vi "VI Tree.vi"   [LabVIEW 2020, in "Agilent 90000 Series.lvlib"]
doc: "This is the instrument driver for the Agilent 90000 and 9000 Series Oscilloscopes. The VI Tree displays all the user-callable VIs of the instrument driver in an organized table."
uses:
  Agilent 90000 Series.lvlib
  Configure/IScan/Configure IScan Trigger (Measurement Limit).vi
  Configure/Measurement/Configure Measurement (Burst Width).vi
  Configure/Trigger/Configure Trigger (Communication).vi
  Data/Read and Save as TDMS (Single Channel).vi
  Data/Read Waveform from TDMS (Unscaled Int8).vi
  Data/Read (Multiple Digital Waveforms).vi
  Data/Low Level/Fetch Measurement (Burst Interval).vi
  Data/Low Level/Fetch (Digital Waveform).vi
  Configure/Measurement/Configure Measurement Characteristics (Eye Pattern).vi
  Data/Read Measurement (Burst Interval).vi
  Configure/Configure Math (Binary Operation).vi
panel:
  # "(c) 2011-2014 National Instruments.  ALL RIGHTS RESERVED."
  # "SEE DIAGRAM\nFOR VI TREE."
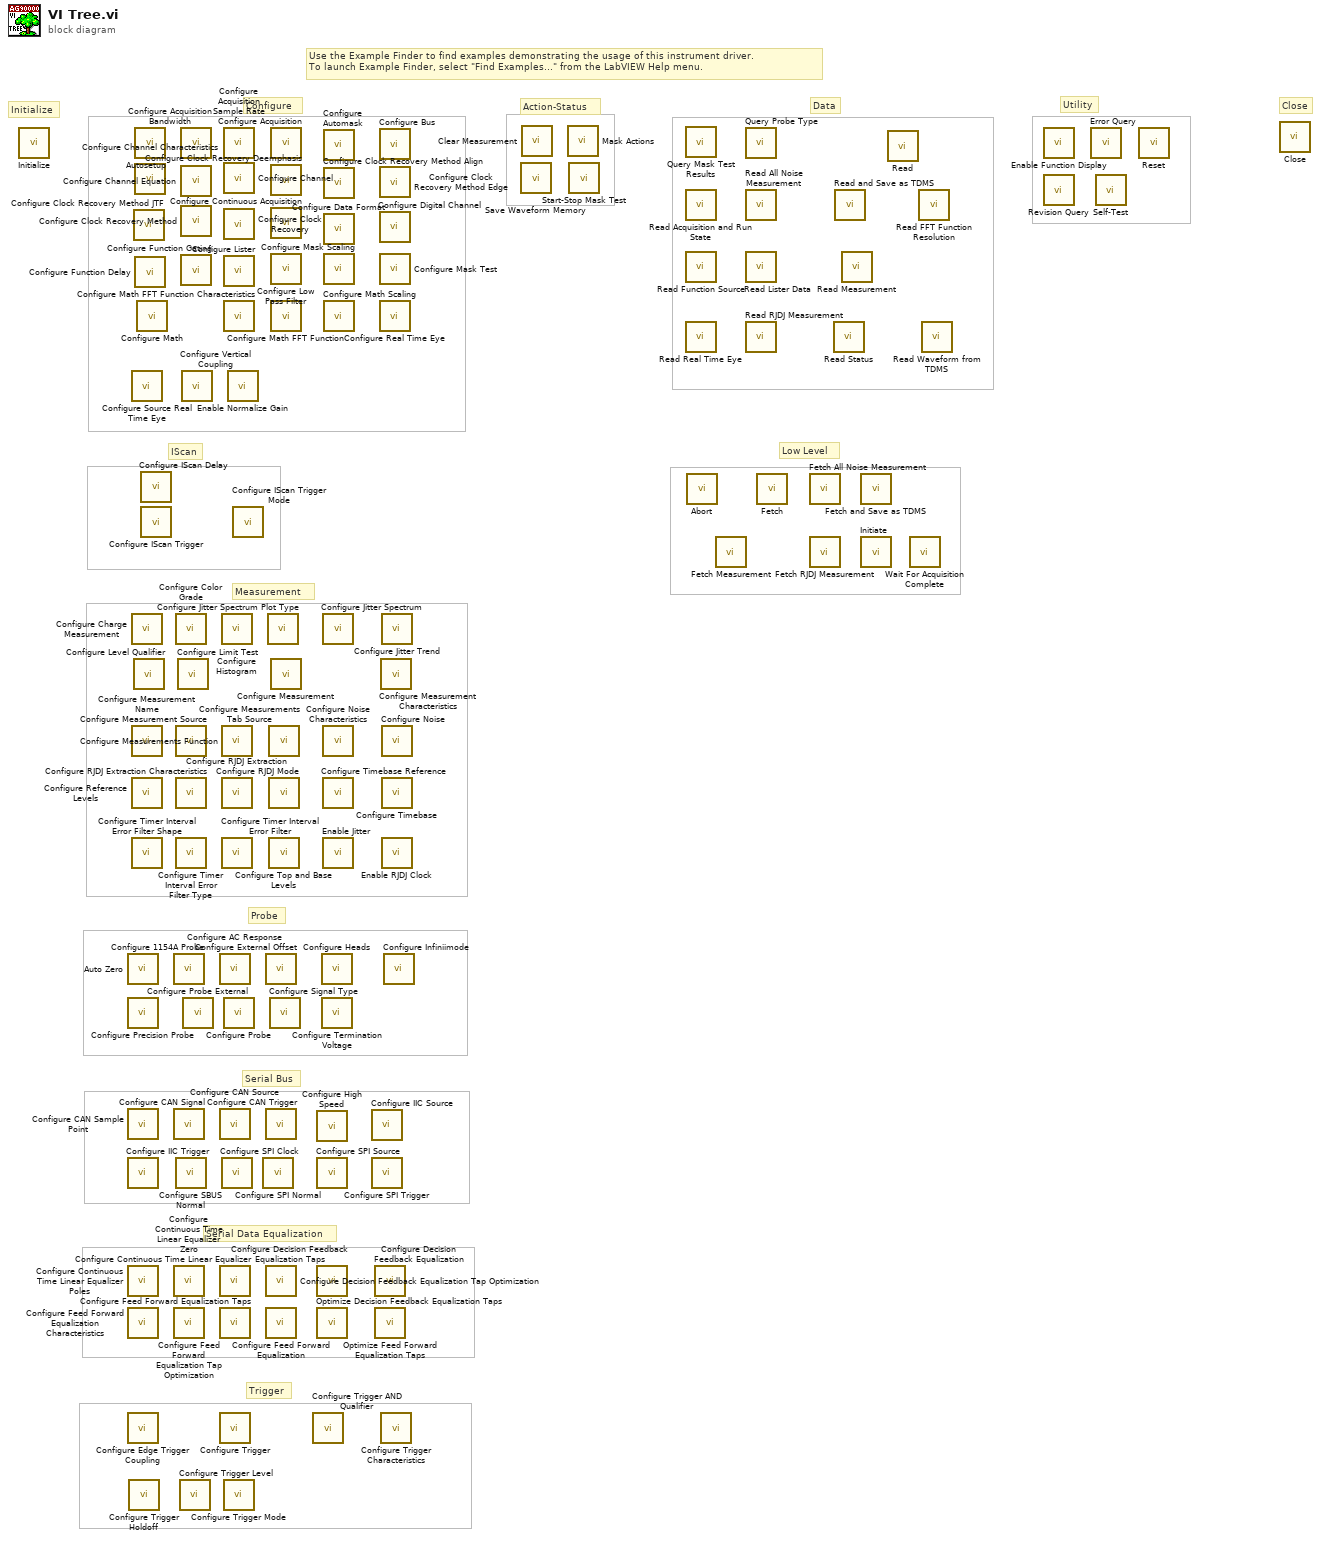
[diagram p0: block diagram]
diagram:
  # "Close"
  # "Utility"
  # "Low Level"
  # "Data"
  # "Trigger"
  # "Serial Data Equalization"
  # "Serial Bus"
  # "Probe"
  # "Measurement"
  # "IScan"
  # "Configure"
  # "Action-Status"
  # "Initialize"
  # "Use the Example Finder to find examples demonstrating the usage of this instrument driver.\nTo launch Example Finder, select \"Find Examples...\" from the LabVIEW Help menu."
  n1 = call "Initialize.vi"() -> ()  [unwired: 9 in, 3 out]
  n2 = call "Auto Zero.vi"() -> ()  [unwired: 10 in, 2 out]
  n3 = call "Configure Precision Probe.vi"() -> ()  [unwired: 14 in, 2 out]
  n4 = call "Configure CAN Sample Point.vi"() -> ()  [unwired: 10 in, 2 out]
  n5 = call "Configure IIC Trigger.vi"() -> ()  [unwired: 10 in, 2 out]
  n6 = call "Configure Continuous Time Linear Equalizer Poles.vi"() -> ()  [unwired: 10 in, 2 out]
  n7 = call "Configure Feed Forward Equalization Characteristics.vi"() -> ()  [unwired: 10 in, 2 out]
  n8 = call "Configure Edge Trigger Coupling.vi"() -> ()  [unwired: 14 in, 2 out]
  n9 = call "Configure Trigger Holdoff.vi"() -> ()  [unwired: 10 in, 2 out]
  n10 = call "Configure Source Real Time Eye.vi"() -> ()  [unwired: 10 in, 2 out]
  n11 = call "Configure Charge Measurement.vi"() -> ()  [unwired: 10 in, 2 out]
  n12 = call "Configure Measurement Name.vi"() -> ()  [unwired: 10 in, 2 out]
  n13 = call "Configure Reference Levels.vi"() -> ()  [unwired: 10 in, 2 out]
  n14 = call "Configure Timer Interval Error Filter Shape.vi"() -> ()  [unwired: 10 in, 2 out]
  n15 = call "Configure Clock Recovery Method JTF.vi"() -> ()  [unwired: 14 in, 2 out]
  n16 = call "Configure Level Qualifier.vi"() -> ()  [unwired: 10 in, 2 out]
  n17 = call "Autosetup.vi"() -> ()  [unwired: 10 in, 2 out]
  n18 = call "Configure Channel Characteristics.vi"() -> ()  [unwired: 10 in, 2 out]
  n19 = call "Configure Function Delay.vi"() -> ()  [unwired: 10 in, 2 out]
  n20 = call-poly "Configure Math.vi"() -> ()  [unwired: 14 in, 2 out]
  n21 = call "Configure IScan Delay.vi"() -> ()  [unwired: 10 in, 2 out]
  n22 = call-poly "Configure IScan Trigger.vi"() -> ()  [unwired: 14 in, 2 out]
  n23 = call "Configure 1154A Probe.vi"() -> ()  [unwired: 10 in, 2 out]
  n24 = call "Configure CAN Signal.vi"() -> ()  [unwired: 10 in, 2 out]
  n25 = call "Configure Continuous Time Linear Equalizer Zero.vi"() -> ()  [unwired: 10 in, 2 out]
  n26 = call "Configure Feed Forward Equalization Tap Optimization.vi"() -> ()  [unwired: 10 in, 2 out]
  n27 = call "Configure Color Grade.vi"() -> ()  [unwired: 14 in, 2 out]
  n28 = call "Configure Measurement Source.vi"() -> ()  [unwired: 10 in, 2 out]
  n29 = call "Configure RJDJ Extraction Characteristics.vi"() -> ()  [unwired: 14 in, 2 out]
  n30 = call "Configure Timer Interval Error Filter Type.vi"() -> ()  [unwired: 14 in, 2 out]
  n31 = call "Configure SBUS Normal.vi"() -> ()  [unwired: 10 in, 2 out]
  n32 = call "Configure Limit Test.vi"() -> ()  [unwired: 10 in, 2 out]
  n33 = call "Configure Trigger Level.vi"() -> ()  [unwired: 10 in, 2 out]
  n34 = call "Configure Acquisition Bandwidth.vi"() -> ()  [unwired: 10 in, 2 out]
  n35 = call "Configure Channel Equation.vi"() -> ()  [unwired: 10 in, 2 out]
  n36 = call "Configure Clock Recovery Method.vi"() -> ()  [unwired: 14 in, 2 out]
  n37 = call "Configure Function Gating.vi"() -> ()  [unwired: 10 in, 2 out]
  n38 = call "Configure Vertical Coupling.vi"() -> ()  [unwired: 10 in, 2 out]
  n39 = call "Configure Probe External.vi"() -> ()  [unwired: 10 in, 2 out]
  n40 = call "Configure AC Response.vi"() -> ()  [unwired: 10 in, 2 out]
  n41 = call "Configure CAN Source.vi"() -> ()  [unwired: 10 in, 2 out]
  n42 = call "Configure Continuous Time Linear Equalizer.vi"() -> ()  [unwired: 14 in, 2 out]
  n43 = call "Configure Feed Forward Equalization Taps.vi"() -> ()  [unwired: 10 in, 2 out]
  n44 = call-poly "Configure Trigger.vi"() -> ()  [unwired: 14 in, 2 out]
  n45 = call "Configure Histogram.vi"() -> ()  [unwired: 14 in, 2 out]
  n46 = call "Configure Measurements Function.vi"() -> ()  [unwired: 10 in, 2 out]
  n47 = call "Configure RJDJ Extraction.vi"() -> ()  [unwired: 14 in, 2 out]
  n48 = call "Configure Timer Interval Error Filter.vi"() -> ()  [unwired: 14 in, 2 out]
  n49 = call "Configure SPI Clock.vi"() -> ()  [unwired: 10 in, 2 out]
  n50 = call "Configure Acquisition Sample Rate.vi"() -> ()  [unwired: 10 in, 2 out]
  n51 = call "Configure Channel.vi"() -> ()  [unwired: 10 in, 2 out]
  n52 = call "Configure Clock Recovery.vi"() -> ()  [unwired: 10 in, 2 out]
  n53 = call "Configure Lister.vi"() -> ()  [unwired: 10 in, 2 out]
  n54 = call "Configure Math FFT Function Characteristics.vi"() -> ()  [unwired: 10 in, 2 out]
  n55 = call "Configure Probe.vi"() -> ()  [unwired: 10 in, 2 out]
  n56 = call "Configure Trigger Mode.vi"() -> ()  [unwired: 14 in, 2 out]
  n57 = call "Enable Normalize Gain.vi"() -> ()  [unwired: 10 in, 2 out]
  n58 = call "Configure IScan Trigger Mode.vi"() -> ()  [unwired: 10 in, 2 out]
  n59 = call "Configure SPI Normal.vi"() -> ()  [unwired: 10 in, 2 out]
  n60 = call "Configure External Offset.vi"() -> ()  [unwired: 10 in, 2 out]
  n61 = call "Configure CAN Trigger.vi"() -> ()  [unwired: 14 in, 2 out]
  n62 = call "Configure Decision Feedback Equalization Tap Optimization.vi"() -> ()  [unwired: 10 in, 2 out]
  n63 = call "Configure Feed Forward Equalization.vi"() -> ()  [unwired: 14 in, 2 out]
  n64 = call "Configure Jitter Spectrum Plot Type.vi"() -> ()  [unwired: 10 in, 2 out]
  n65 = call "Configure Measurements Tab Source.vi"() -> ()  [unwired: 10 in, 2 out]
  n66 = call "Configure RJDJ Mode.vi"() -> ()  [unwired: 10 in, 2 out]
  n67 = call "Configure Top and Base Levels.vi"() -> ()  [unwired: 14 in, 2 out]
  n68 = call "Configure Signal Type.vi"() -> ()  [unwired: 10 in, 2 out]
  n69 = call "Configure Acquisition.vi"() -> ()  [unwired: 14 in, 2 out]
  n70 = call "Configure Clock Recovery Deemphasis.vi"() -> ()  [unwired: 10 in, 2 out]
  n71 = call "Configure Continuous Acquisition.vi"() -> ()  [unwired: 10 in, 2 out]
  n72 = call "Configure Low Pass Filter.vi"() -> ()  [unwired: 10 in, 2 out]
  n73 = call "Configure Math FFT Function.vi"() -> ()  [unwired: 10 in, 2 out]
  n74 = call-poly "Configure Measurement.vi"() -> ()  [unwired: 14 in, 2 out]
  n75 = call "Configure Trigger AND Qualifier.vi"() -> ()  [unwired: 14 in, 2 out]
  n76 = call "Configure High Speed.vi"() -> ()  [unwired: 14 in, 2 out]
  n77 = call "Configure SPI Source.vi"() -> ()  [unwired: 10 in, 2 out]
  n78 = call "Configure Decision Feedback Equalization Taps.vi"() -> ()  [unwired: 10 in, 2 out]
  n79 = call "Optimize Decision Feedback Equalization Taps.vi"() -> ()  [unwired: 10 in, 2 out]
  n80 = call "Configure Heads.vi"() -> ()  [unwired: 10 in, 2 out]
  n81 = call "Configure Termination Voltage.vi"() -> ()  [unwired: 10 in, 2 out]
  n82 = call "Configure Jitter Spectrum.vi"() -> ()  [unwired: 14 in, 2 out]
  n83 = call "Configure Noise Characteristics.vi"() -> ()  [unwired: 10 in, 2 out]
  n84 = call "Configure Timebase Reference.vi"() -> ()  [unwired: 10 in, 2 out]
  n85 = call "Enable Jitter.vi"() -> ()  [unwired: 10 in, 2 out]
  n86 = call "Configure Automask.vi"() -> ()  [unwired: 10 in, 2 out]
  n87 = call "Configure Clock Recovery Method Align.vi"() -> ()  [unwired: 10 in, 2 out]
  n88 = call "Configure Data Format.vi"() -> ()  [unwired: 10 in, 2 out]
  n89 = call "Configure Mask Scaling.vi"() -> ()  [unwired: 10 in, 2 out]
  n90 = call "Configure Math Scaling.vi"() -> ()  [unwired: 10 in, 2 out]
  n91 = call "Configure IIC Source.vi"() -> ()  [unwired: 10 in, 2 out]
  n92 = call "Configure SPI Trigger.vi"() -> ()  [unwired: 10 in, 2 out]
  n93 = call "Configure Decision Feedback Equalization.vi"() -> ()  [unwired: 14 in, 2 out]
  n94 = call "Optimize Feed Forward Equalization Taps.vi"() -> ()  [unwired: 10 in, 2 out]
  n95 = call "Configure Bus.vi"() -> ()  [unwired: 10 in, 2 out]
  n96 = call "Configure Clock Recovery Method Edge.vi"() -> ()  [unwired: 10 in, 2 out]
  n97 = call "Configure Digital Channel.vi"() -> ()  [unwired: 10 in, 2 out]
  n98 = call "Configure Mask Test.vi"() -> ()  [unwired: 14 in, 2 out]
  n99 = call "Configure Real Time Eye.vi"() -> ()  [unwired: 14 in, 2 out]
  n100 = call-poly "Configure Measurement Characteristics.vi"() -> ()  [unwired: 14 in, 2 out]
  n101 = call "Configure Trigger Characteristics.vi"() -> ()  [unwired: 14 in, 2 out]
  n102 = call "Configure Jitter Trend.vi"() -> ()  [unwired: 14 in, 2 out]
  n103 = call "Configure Noise.vi"() -> ()  [unwired: 10 in, 2 out]
  n104 = call "Configure Timebase.vi"() -> ()  [unwired: 10 in, 2 out]
  n105 = call "Enable RJDJ Clock.vi"() -> ()  [unwired: 10 in, 2 out]
  n106 = call "Configure Infiniimode.vi"() -> ()  [unwired: 10 in, 2 out]
  n107 = call "Save Waveform Memory.vi"() -> ()  [unwired: 10 in, 2 out]
  n108 = call "Clear Measurement.vi"() -> ()  [unwired: 10 in, 2 out]
  n109 = call "Mask Actions.vi"() -> ()  [unwired: 10 in, 2 out]
  n110 = call "Start-Stop Mask Test.vi"() -> ()  [unwired: 10 in, 2 out]
  n111 = call "Query Mask Test Results.vi"() -> ()  [unwired: 6 in, 6 out]
  n112 = call "Read Acquisition and Run State.vi"() -> ()  [unwired: 8 in, 4 out]
  n113 = call "Read Function Source.vi"() -> ()  [unwired: 8 in, 4 out]
  n114 = call "Read Real Time Eye.vi"() -> ()  [unwired: 8 in, 4 out]
  n115 = call "Abort.vi"() -> ()  [unwired: 10 in, 2 out]
  n116 = call-poly "Fetch Measurement.vi"() -> ()  [unwired: 13 in, 3 out]
  n117 = call "Query Probe Type.vi"() -> ()  [unwired: 9 in, 3 out]
  n118 = call "Read All Noise Measurement.vi"() -> ()  [unwired: 6 in, 10 out]
  n119 = call "Read Lister Data.vi"() -> ()  [unwired: 9 in, 3 out]
  n120 = call "Read RJDJ Measurement.vi"() -> ()  [unwired: 5 in, 11 out]
  n121 = call-poly "Fetch.vi"() -> ()  [unwired: 13 in, 3 out]
  n122 = call "Fetch All Noise Measurement.vi"() -> ()  [unwired: 6 in, 10 out]
  n123 = call "Fetch RJDJ Measurement.vi"() -> ()  [unwired: 5 in, 11 out]
  n124 = call "Read Status.vi"() -> ()  [unwired: 9 in, 3 out]
  n125 = call-poly "Read and Save as TDMS.vi"() -> ()  [unwired: 12 in, 4 out]
  n126 = call-poly "Read Measurement.vi"() -> ()  [unwired: 13 in, 3 out]
  n127 = call "Fetch and Save as TDMS.vi"() -> ()  [unwired: 12 in, 4 out]
  n128 = call "Initiate.vi"() -> ()  [unwired: 10 in, 2 out]
  n129 = call-poly "Read.vi"() -> ()  [unwired: 13 in, 3 out]
  n130 = call "Wait For Acquisition Complete.vi"() -> ()  [unwired: 10 in, 2 out]
  n131 = call "Read FFT Function Resolution.vi"() -> ()  [unwired: 9 in, 3 out]
  n132 = call-poly "Read Waveform from TDMS.vi"() -> ()  [unwired: 12 in, 4 out]
  n133 = call "Enable Function Display.vi"() -> ()  [unwired: 10 in, 2 out]
  n134 = call "Revision Query.vi"() -> ()  [unwired: 8 in, 4 out]
  n135 = call "Error Query.vi"() -> ()  [unwired: 8 in, 4 out]
  n136 = call "Self-Test.vi"() -> ()  [unwired: 8 in, 4 out]
  n137 = call "Reset.vi"() -> ()  [unwired: 10 in, 2 out]
  n138 = call "Close.vi"() -> ()  [unwired: 11 in, 1 out]
